vi "Dust_Type_Query.vi"(8 "error in (no error)":errorcluster) -> (0 "error out":errorcluster, 3 "Dust Type Array":T1[](array[typedef]))   [LabVIEW 2015]
doc: "Sub-vi of Search_dust_name and Search_Dust_Type. Searches the dust_type table for all rows for which the dust_name contains the given string. An empty string (default) returns all rows from the dust_type table."
uses:
  User Interface/Controls/Dust_list.ctl
  <vilib>/addons/database/_DB Variant To Data/Database Variant To Data.xnode
panel:
  out "Query in Standard Format":string
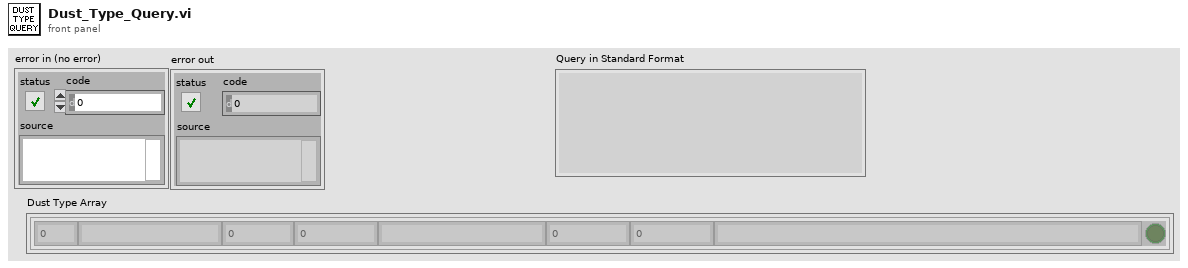
[diagram p1: front panel]
types:
  T1 = typedef "Dust_list.ctl" = cluster{"id_dust_type":i32, "dust_name":string, "dust_type":i32, "batch_no":i32, "dust_density":dbl, "source_weight":dbl, "size":string, "bottle_weight":dbl, "dust_mass":dbl, "comments":string, "Shoots?":bool}
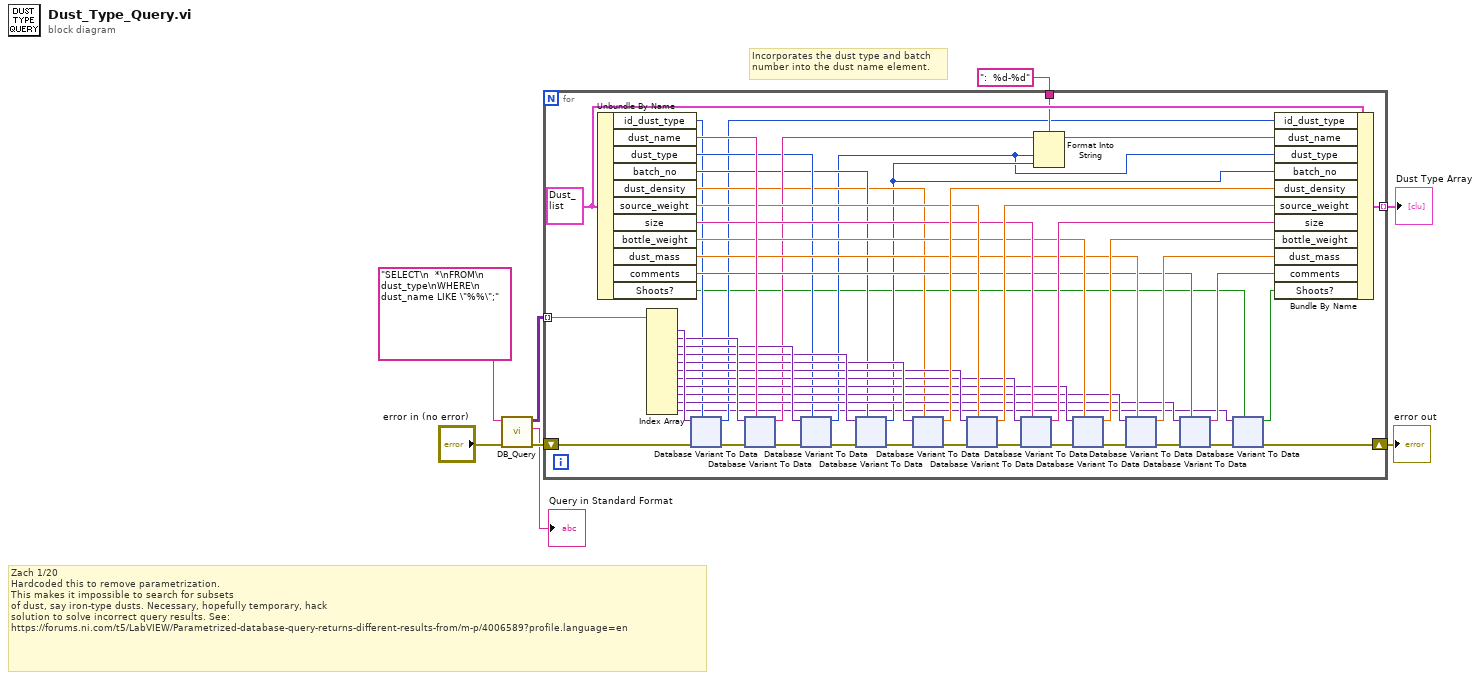
[diagram p0: block diagram]
diagram:
  # "Zach 1/20\nHardcoded this to remove parametrization. \nThis makes it impossible to search for subsets\nof dust, say iron-type dusts. Necessary, hopefully temporary, hack\nsolution to solve incorrect query results. See:\nhttps://forums.ni.com/t5/LabVIEW/Parametrized-database-query-returns-different-results-from/m-p/4006589?profile.language=en"
  # "Incorporates the dust type and batch\nnumber into the dust name element."
  n1 = call "DB_Query.vi"("error in (no error)"="error in (no error)", "Parameterized Query"="SELECT\n  *\nFROM\n  dust_type\nWHERE\n  dust_name LIKE \"%%\";") -> ("error out"=w7:errorcluster, "Query in Standard Format"=→"Query in Standard Format":string, "Results"=w5:variant[][])  [unwired: 7 in]
  n2 = for {
    shift-right: [w9] -> w6
    shift-left: w7 -> [w55]
    tunnel: w5 -> [w58] mode=indexing
    tunnel: [w56] -> w4 mode=indexing
    tunnel: ":  %d-%d" -> [w48]
    w57 = T1 {"id_dust_type"=0, "dust_name"="", "dust_type"=0, "batch_no"=0, "dust_density"=0.0, "source_weight"=0.0, "size"="", "bottle_weight"=0.0, "dust_mass"=0.0, "comments"="", "Shoots?"=FALSE} ("Cluster")
    n3 = Unbundle By Name(w57) -> ("id_dust_type"=w15:i32, "dust_name"=w51:string, "dust_type"=w20:i32, "batch_no"=w19:i32, "dust_density"=w18:dbl, "source_weight"=w41:dbl, "size"=w36:string, "bottle_weight"=w33:dbl, "dust_mass"=w28:dbl, "comments"=w24:string, "Shoots?"=w11:bool)
    n4 = Index Array(array=w58) -> (element #1=w54:variant, element #2=w52:variant, element #3=w49:variant, element #4=w46:variant, element #5=w44:variant, element #6=w40:variant, element #7=w37:variant, element #8=w32:variant, element #9=w29:variant, element #10=w25:variant, element #11=w12:variant)  [unwired: 11 in]
    n5 = xnode "Database Variant To Data"("database variant"=w54, "error in (no error)"=w55, "type"=w15) -> ("data"=w14:i32, "error out"=w53:errorcluster)
    n6 = xnode "Database Variant To Data"("database variant"=w52, "error in (no error)"=w53, "type"=w51) -> ("data"=w22:string, "error out"=w50:errorcluster)
    n7 = xnode "Database Variant To Data"("database variant"=w49, "error in (no error)"=w50, "type"=w20) -> ("data"=w16:i32, "error out"=w47:errorcluster)
    n8 = xnode "Database Variant To Data"("database variant"=w46, "error in (no error)"=w47, "type"=w19) -> ("data"=w17:i32, "error out"=w45:errorcluster)
    n9 = xnode "Database Variant To Data"("database variant"=w44, "error in (no error)"=w45, "type"=w18) -> ("data"=w43:dbl, "error out"=w42:errorcluster)
    n10 = xnode "Database Variant To Data"("database variant"=w40, "error in (no error)"=w42, "type"=w41) -> ("data"=w38:dbl, "error out"=w39:errorcluster)
    n11 = xnode "Database Variant To Data"("database variant"=w37, "error in (no error)"=w39, "type"=w36) -> ("data"=w35:string, "error out"=w34:errorcluster)
    n12 = Format Into String(format string=w48, initial string=w22, w16, w17) -> (resulting string=w21:string)  [unwired: 1 in, 1 out]
    n13 = xnode "Database Variant To Data"("database variant"=w32, "error in (no error)"=w34, "type"=w33) -> ("data"=w31:dbl, "error out"=w30:errorcluster)
    n14 = xnode "Database Variant To Data"("database variant"=w29, "error in (no error)"=w30, "type"=w28) -> ("data"=w27:dbl, "error out"=w26:errorcluster)
    n15 = xnode "Database Variant To Data"("database variant"=w25, "error in (no error)"=w26, "type"=w24) -> ("data"=w23:string, "error out"=w13:errorcluster)
    n16 = xnode "Database Variant To Data"("database variant"=w12, "error in (no error)"=w13, "type"=w11) -> ("data"=w10:bool, "error out"=w9:errorcluster)
    n17 = Bundle By Name(cluster=w57, "id_dust_type"=w14, "dust_name"=w21, "dust_type"=w16, "batch_no"=w17, "dust_density"=w43, "source_weight"=w38, "size"=w35, "bottle_weight"=w31, "dust_mass"=w27, "comments"=w23, "Shoots?"=w10) -> (w56:T1)
  }
  "error out" <- w6
  "Dust Type Array" <- w4
